vi "Get Connector Pane Ref.vi"(0 "VI Reference":refnum<vi>, 1 "error in (no error)":errorcluster) -> (2 "VI Reference out":refnum<vi>, 3 "Connector Pane":refnum<vi>, 4 "error out":errorcluster)   [LabVIEW 2012, in "Scripting Tools.lvlib"]
doc: "Get a reference to the connector pane of a vi"
uses:
  Scripting Tools.lvlib
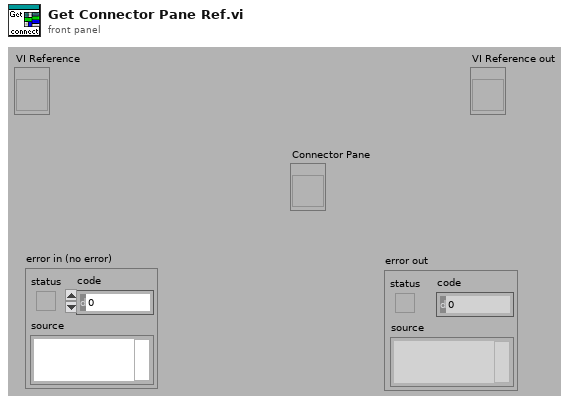
[diagram p1: front panel]
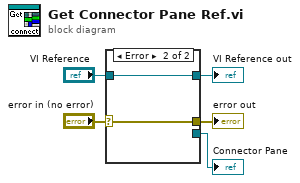
[diagram p0: block diagram]
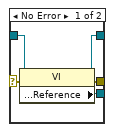
[diagram p2: hidden frame]
diagram:
  n1 = case shown="Error" "error in (no error)" {
    selector: "error in (no error)" -> [w6 w12]
    tunnel: "VI Reference" -> [w10 w11]
    tunnel: [w9 w11] -> w4
    tunnel: [w8 _] -> w3
    tunnel: [w7 w12] -> w2
    frame No Error {
      n2 = property class="VI"(reference=w10, error in=w6) -> (reference out=w9:refnum<vi>, error out=w7:errorcluster, "Connector Pane:Reference"=w8:refnum<vi>)
    }
    frame Error {
    }
  }
  "VI Reference out" <- w4
  "error out" <- w2
  "Connector Pane" <- w3
